vi "[BLE Test] ble_read_write_characteristics.vi"() -> ()   [LabVIEW 2015]
uses:
  Lib_Bled112 toolkit/type_def/connection_status_bundle.ctl
  Lib_Bled112 toolkit/type_def/address_type.ctl
  Lib_Bled112 toolkit/type_def/message_type.ctl
  Lib_Bled112 toolkit/type_def/message_class.ctl
  Lib_Bled112 toolkit/ble_functions/ble_write_by_handle_uint8array.vi
panel:
  out "Rx Packet Structure":T1={"Message Type (Response)"=128, "Payload length"=0, "Command Class (System)"=1, "Message ID"=0, "Connection handle"=0, "Attribute handle"=0, "Attribute type"=1, "Attribute value (data)"=[]} {"Attribute type" format="%02x" items=["read", "notify", "indicate", "read_by_type", "read_blob", "indicate_rsp_req"]; "Attribute value (data)" format="%02x"; "Attribute handle" format="%04x"; "Connection handle" format="%02x"; "Message ID" format="%02x"; "Message Type (Response)" format="%02x" items=["Command / Response"=0, "Event"=128]; "Command Class (System)" format="%02x" items=["System", "Persistent Store", "Attribute database", "Connection", "Attribute client", "Security Manager", "Generic Access Profile", "Hardware"]}
  out "Packet Detect":bool=TRUE
  out "Disconnected":bool=TRUE
  out "Scan success?":bool
  out "BLED112 Dongle Info":string="Major: 1, Minor: 3, Patch: 2, Build: 122, LL ver: 3, Protocol ver: 1 and HW ver: 3  "
  out "그래프 타이머 값 1":u32=9582380
  out "CDC(PCAP02) Graph":waveform(sgl)[](graph)=[{"t0"=timestamp(3554331896.4574084 s since 1904-01-01), "dt"=0.03, "Y"=[1.0007696]}, {"t0"=timestamp(3554331896.4574084 s since 1904-01-01), "dt"=0.03, "Y"=[1.0004687]}]
  out "Working Time(H:M:S)":string="00:01:58"
  out "ms 타이머 값 2":u32=9464045
  in  "Device List":i32(listbox)=2
  out "Rx packet Interval graph":u32(graph)=30
  in  "Program Exit":bool=TRUE
  out "부분배열 2":u8[](array[numeric])=[253, 79, 255, 49, 255, 79, 255, 60, 255, 209, 65, 123, 0, 0, 0, 0, 0, 0, 0, 0] format="%x"
  out "Data-IMU":dbl=-3.014375 format="%.10f"
  out "Hex-IMU":i16=-689 format="%x"
  out "웨이브폼 차트-IMU":dbl(graph)=-3.014375
  in  "Index-IMU ch.":u8(slide)=1 min=1 max=6 step=1 scale=1.0..6.0
  out "Rx OK":bool=TRUE
  out "ms 타이머 값":u32=9582439
  out "Entire-Rx time(ms)":i32=30
  in  "Index-CDC ch.":u8(slide)=1 min=1 max=6 step=1 scale=1.0..6.0
  out "웨이브폼 차트 - CDC":sgl(graph)=1.0007696
  out "Hex-CDC":u32=2098766 format="%x"
  out "Data-CDC":dbl=1.0007696151733398 format="%.10f"
  out "부분배열":u8[](array[numeric])=[32, 6, 78, 32, 3, 215, 32, 6, 110, 32, 71, 249, 32, 115, 92, 32, 30, 38, 1, 0] format="%x"
  in  "Tx 문자열":string="\nBLED112 Test\n"
  in  "Tx Send":bool
  out "Rx Cnt":i32=3775
  in  "Rx Stop":bool=TRUE
  out "Rx 문자열 1":string
  out "Connected":bool
  out "Device Name":string
  out "Address Type":enum16{"Public", "Random"}(ring)=enum."Random"
  out "Handle table":string[][](array[string])
  out "Connection Status":T4 {"Address Type" items=["Public", "Random"]}
  out "Scanning":bool
  in  "Device Connect":bool=TRUE
  out "MAC Address":string="D9:2F:10:92:34:F2"
  in  "COM Bluegiga in":refnum<visa-resource-name>="COM8"
  # "GEN4 1st PP - BLE(Bluetooth Low Energy) Test"
  # "CDC Data"
  # "SCAN"
  # "DEVICES FOUND"
  # "CONNECT"
  # "Introduce the MAC Address and Address Type of the device you want to connect and click in the CONTINUE button"
  # "IMU Data"
  # "Service 0x1800\nCharacteristic 0x2A00\nDevice Name"
  # "READING DEVICE NAME"
  # "Read"
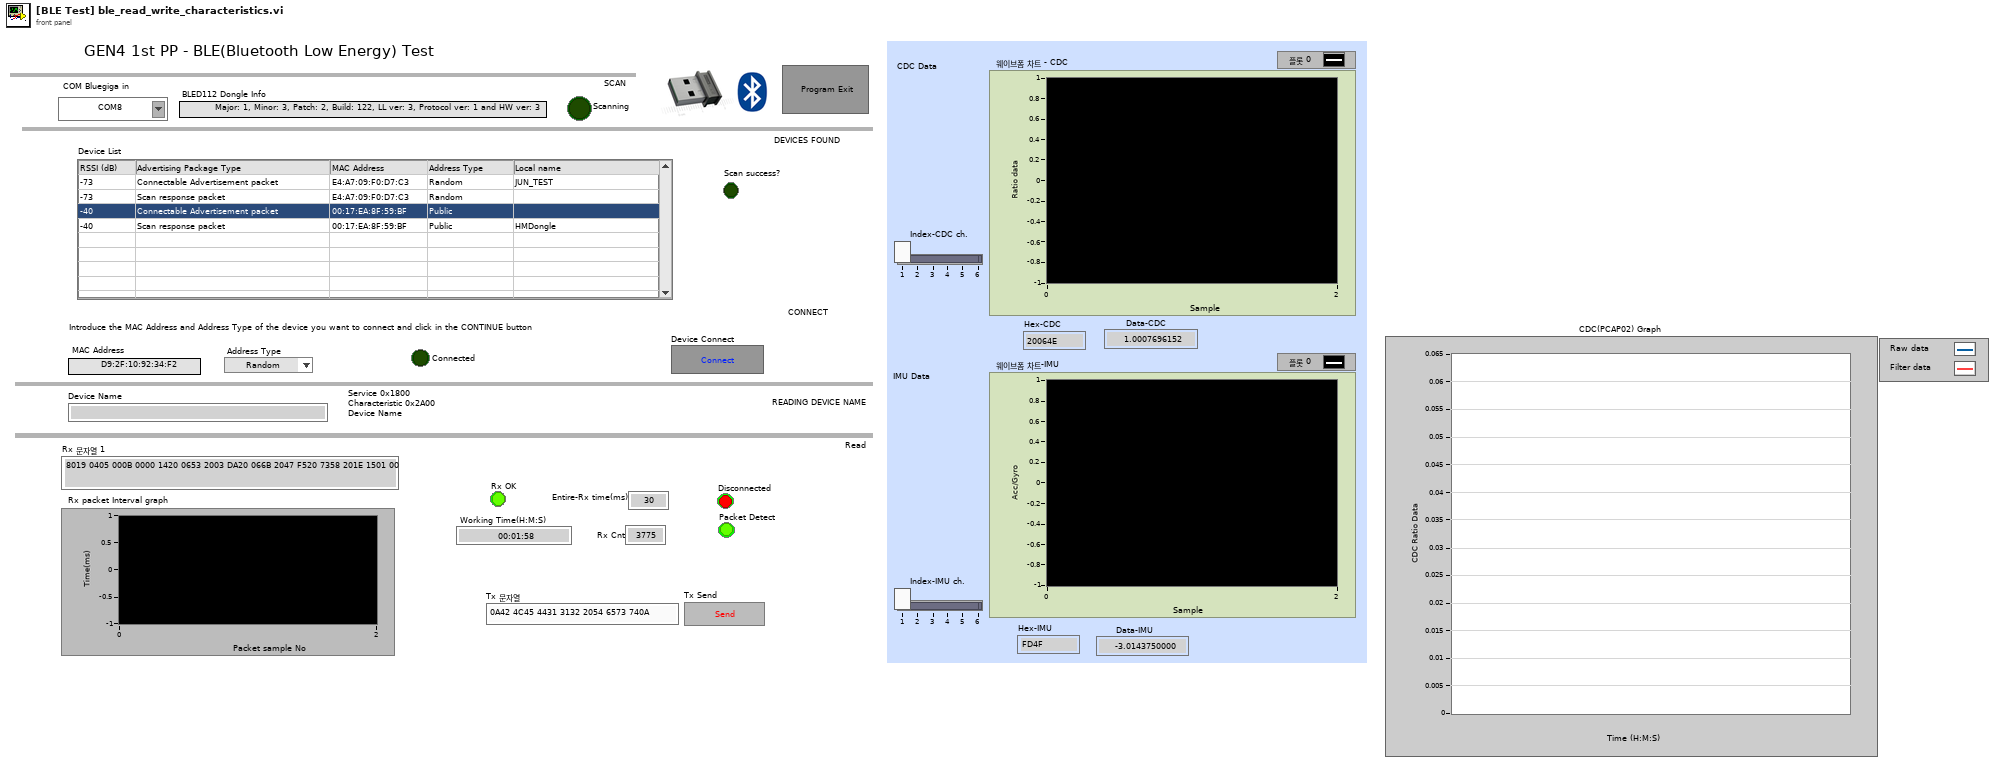
[diagram p1: front panel]
types:
  T1 = typedef "컨트롤-BLED Rx (EVENT-Attribute Client).ctl" = cluster{"Message Type (Response)":T2, "Payload length":u8, "Command Class (System)":T3, "Message ID":u8, "Connection handle":u8, "Attribute handle":u16, "Attribute type":T3, "Attribute value (data)":u8[]}
  T2 = typedef "message_type.ctl" = u8
  T3 = typedef "message_class.ctl" = u8
  T4 = typedef "connection_status_bundle.ctl" = cluster{"MAC Address":string, "cnx handle":u8, "cnx flags":u8, "Address Type":T5, "Connection Interval (ms)":u16, "Timeout(ms)":u16, "Latency":u16, "bonding handle":u8}
  T5 = typedef "address_type.ctl" = u8
  T6 = typedef "컨트롤-BLED Rx (EVENT-Connection status).ctl" = cluster{"Message Type (Response)":T2, "Payload length":u8, "Command Class (System)":T3, "Message ID":u8, "Connection handle":u8, "flags":u8, "Bluetooth address":u8[], "address type":T3, "conn_interval(ms)":dbl, "timeout(ms)":dbl, "latency":u16, "bonding(0xFF)":u8}
  T7 = typedef "컨트롤-BLED Rx (EVENT-Disconnected).ctl" = cluster{"Message Type (Response)":T2, "Payload length":u8, "Command Class (Connection)":T3, "Message ID":u8, "connection":u8, "reason":u16}
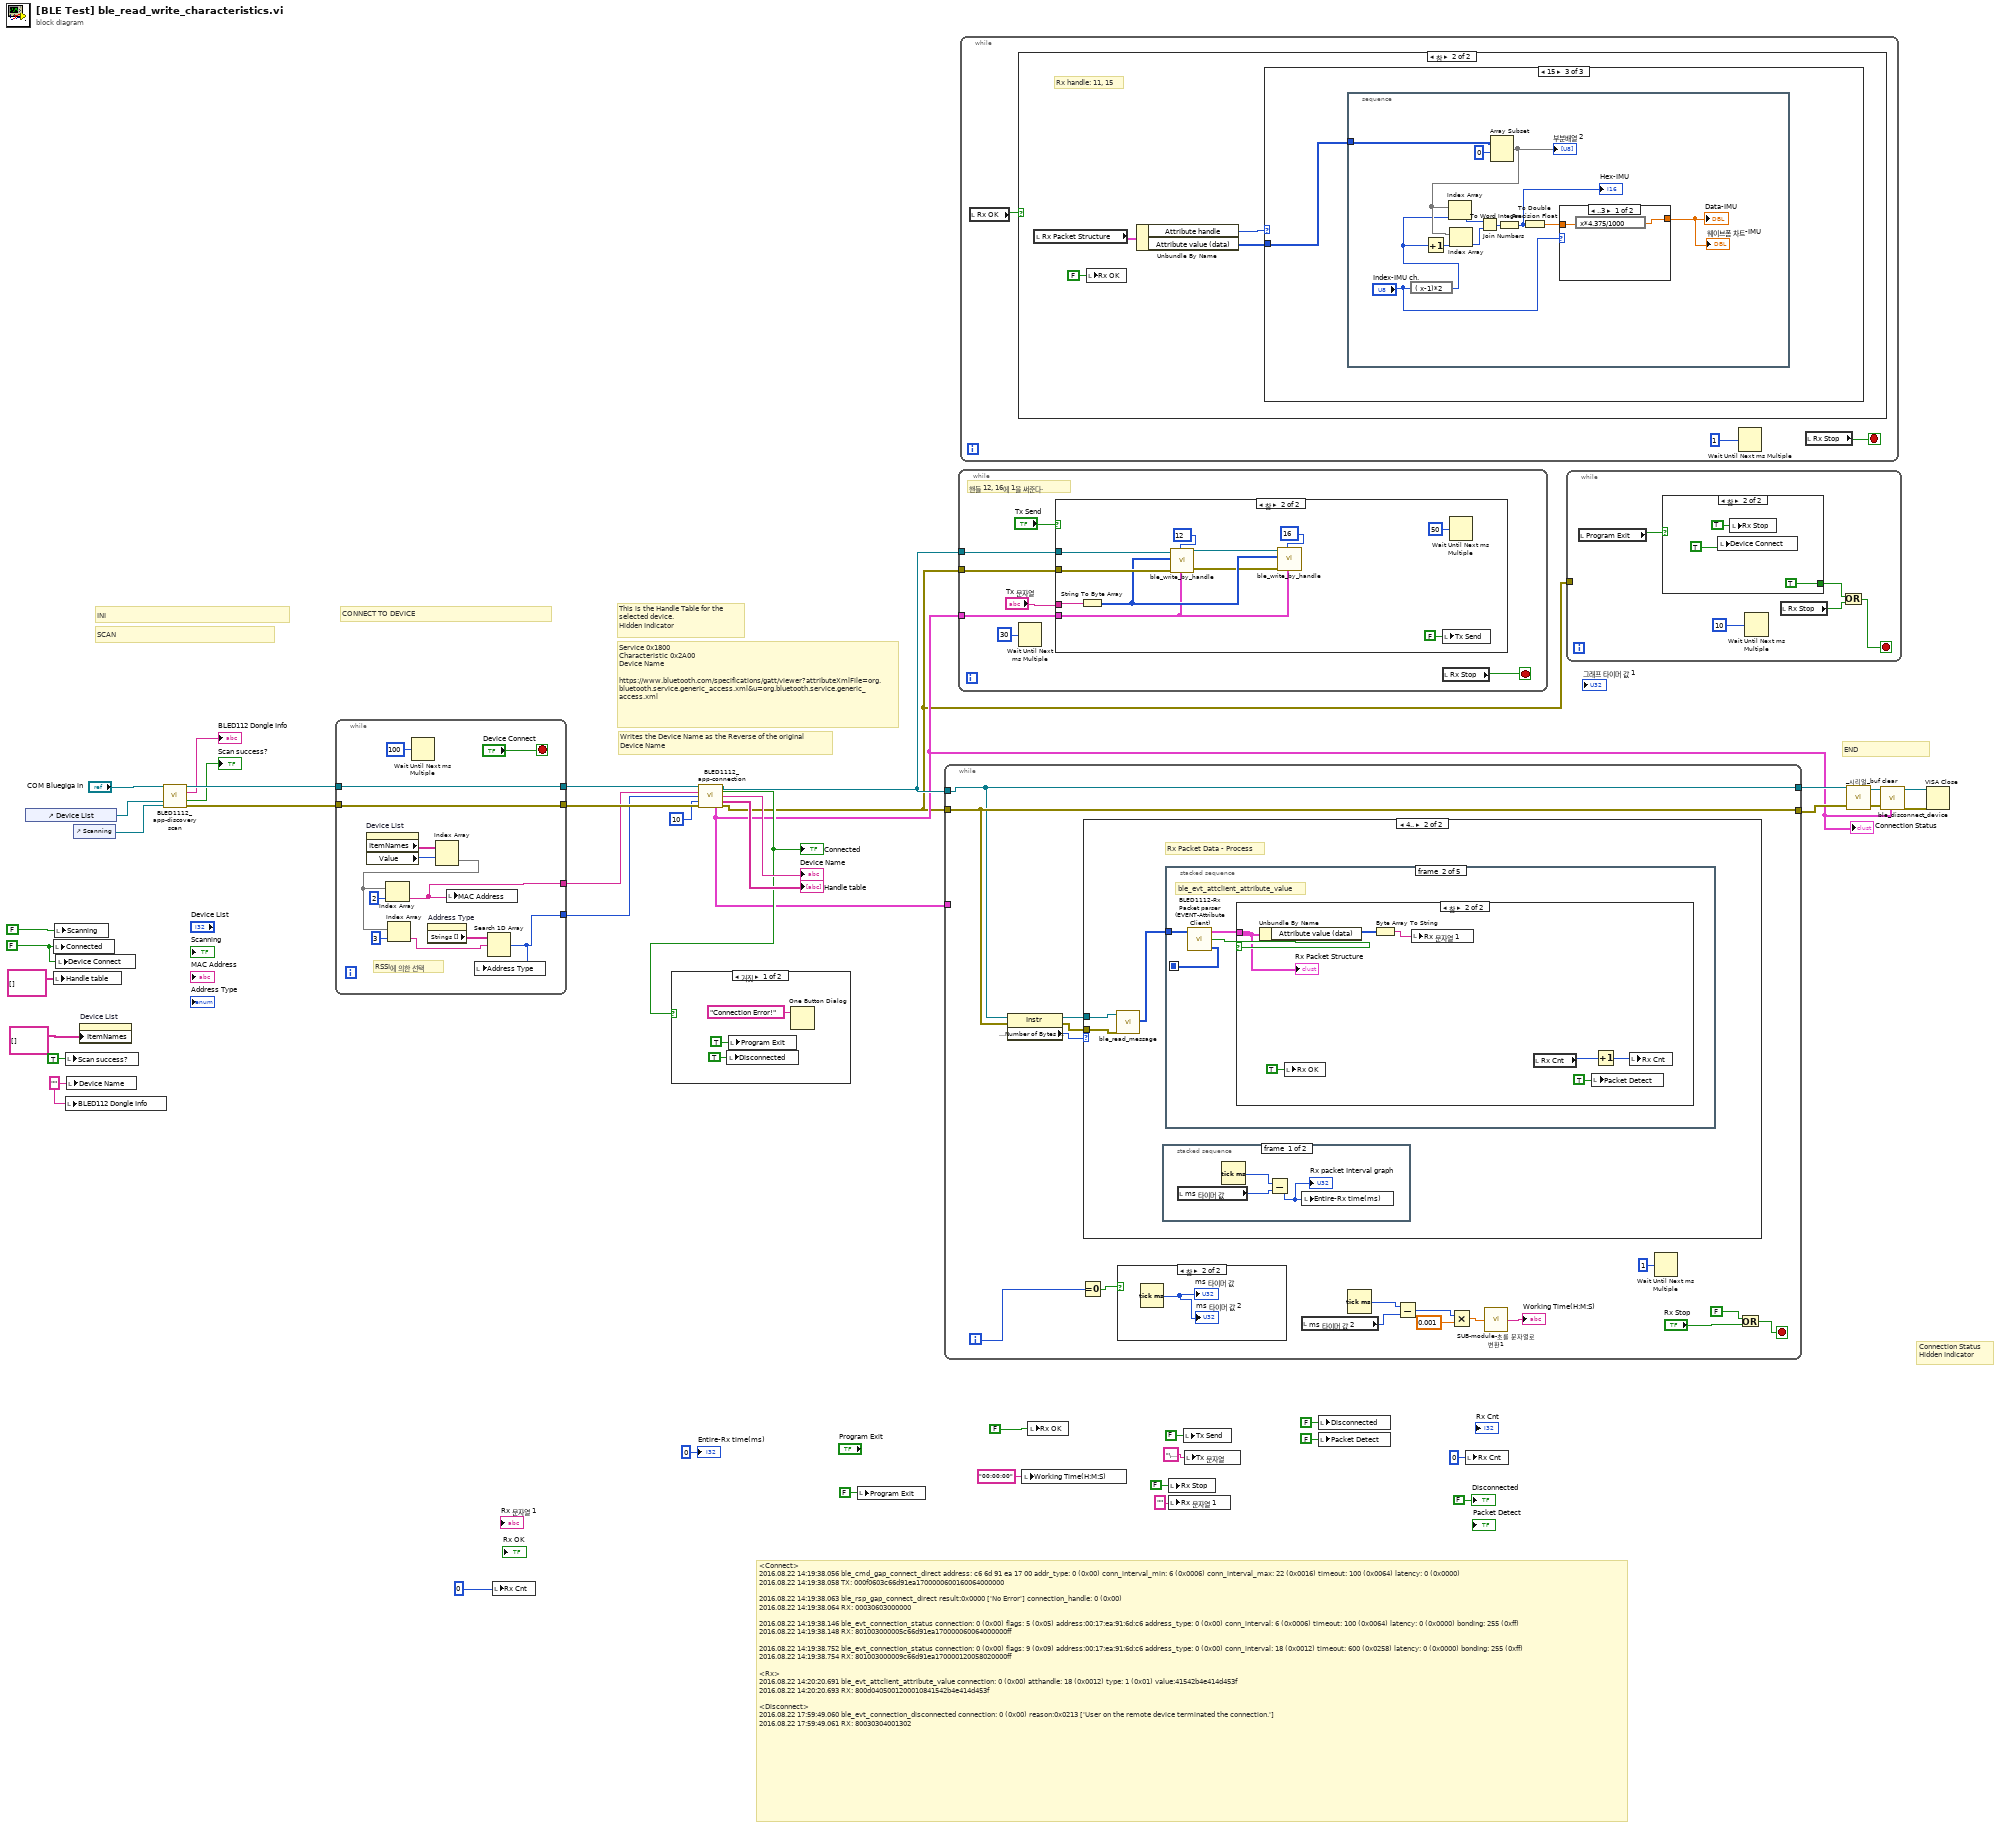
[diagram p0: block diagram]
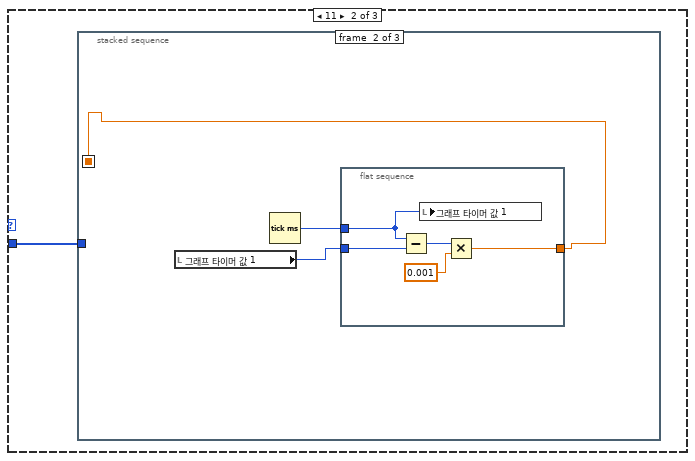
[diagram p7: hidden frame]
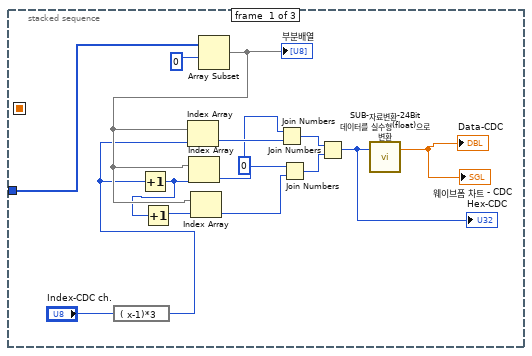
[diagram p8: hidden frame]
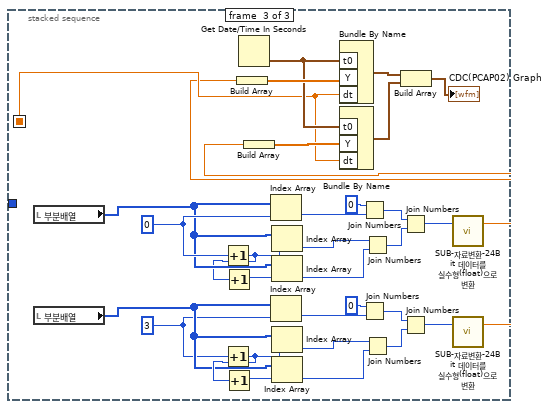
[diagram p9: hidden frame]
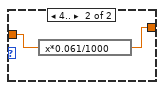
[diagram p10: hidden frame]
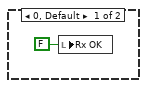
[diagram p11: hidden frame]
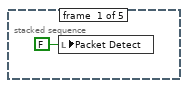
[diagram p12: hidden frame]
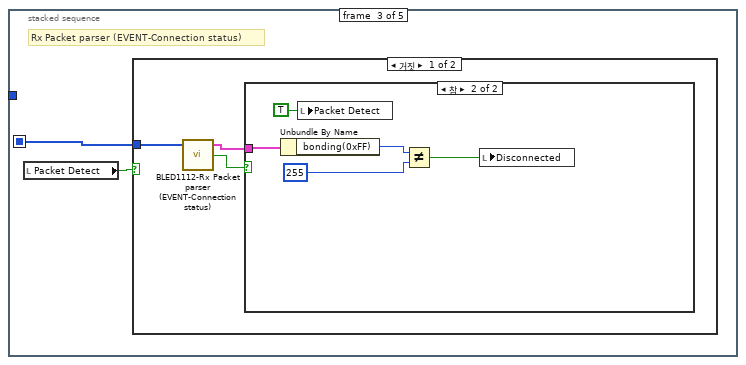
[diagram p14: hidden frame]
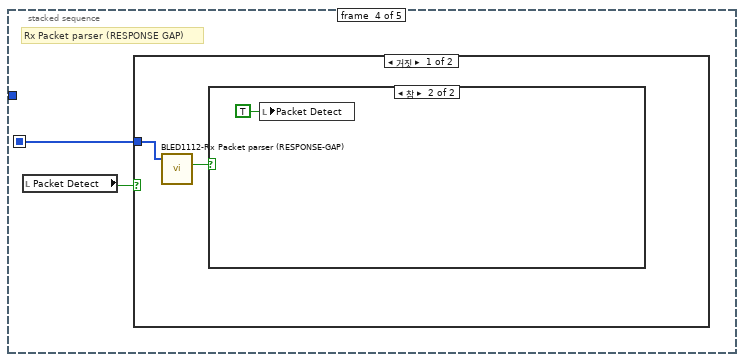
[diagram p17: hidden frame]
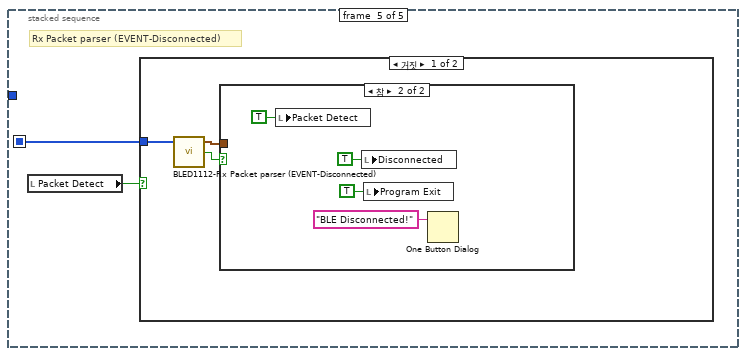
[diagram p20: hidden frame]
diagram:
  w19 = "" ("Device Name")
  w40 = FALSE ("Connected")
  # "<Connect>\n2016.08.22 14:19:38.056 ble_cmd_gap_connect_direct address: c6 6d 91 ea 17 00 addr_type: 0 (0x00) conn_interval_min: 6 (0x0006) conn_interval_max: 22 (0x0016) timeout: 100 (0x0064) latency: 0 (0x0000)\n2016.08.22 14:19:38.058 TX: 000f0603c66d91ea1700000600160064000000\n\n2016.08.22 14:19:38.063 ble_rsp_gap_connect_direct result:0x0000 ['No Error'] connection_handle: 0 (0x00)\n2016.08.22 14:19:38.064 RX: 00030603000000\n\n2016.08.22 14:19:38.146 ble_evt_connection_status connection: 0 (0x00) flags: 5 (0x05) address:00:17:ea:91:6d:c6 address_type: 0 (0x00) conn_interval: 6 (0x0006) timeout: 100 (0x0064) latency: 0 (0x0000) bonding: 255 (0xff)\n2016.08.22 14:19:38.148 RX: 801003000005c66d91ea170000060064000000ff\n\n2016.08.22 14:19:38.752 ble_evt_connection_status connection: 0 (0x00) flags: 9 (0x09) address:00:17:ea:91:6d:c6 address_type: 0 (0x00) conn_interval: 18 (0x0012) timeout: 600 (0x0258) latency: 0 (0x0000) bonding: 255 (0xff)\n2016.08.22 14:19:38.754 RX: 801003000009c66d91ea170000120058020000ff\n\n<Rx>\n2016.08.22 14:20:20.691 ble_evt_attclient_attribute_value connection: 0 (0x00) atthandle: 18 (0x0012) type: 1 (0x01) value:41542b4e414d453f\n2016.08.22 14:20:20.693 RX: 800d0405001200010841542b4e414d453f\n\n<Disconnect>\n2016.08.22 17:59:49.060 ble_evt_connection_disconnected connection: 0 (0x00) reason:0x0213 ['User on the remote device terminated the connection.']\n2016.08.22 17:59:49.061 RX: 80030304001302"
  # "Writes the Device Name as the Reverse of the original\nDevice Name"
  # "Service 0x1800\nCharacteristic 0x2A00\nDevice Name\n\nhttps://www.bluetooth.com/specifications/gatt/viewer?attributeXmlFile=org.bluetooth.service.generic_access.xml&u=org.bluetooth.service.generic_access.xml"
  # "This is the Handle Table for the\nselected device. \nHidden Indicator"
  # "Connection Status\nHidden Indicator"
  # "CONNECT TO DEVICE"
  # "SCAN"
  # "END"
  # "INI"
  n1 = control-ref of="Device List"() -> (w23:refnum<vi>)
  n2 = local write "Connected"(w40) -> ()
  n3 = local write "Handle table"(string[][] [] ("Handle table")) -> ()
  n4 = local write "Scanning"(FALSE ("Scanning")) -> ()
  n5 = local write "Device Connect"(w40) -> ()
  n6 = local write "Scan success?"(TRUE ("Scan success?")) -> ()
  n7 = local write "BLED112 Dongle Info"(w19) -> ()
  n8 = local write "Device Name"(w19) -> ()
  n9 = control-ref of="Scanning"() -> (w22:refnum<vi>)
  n10 = property on="Device List" class="MCListbox (엄격한)"("ItemNames"=string[][] [] ("Devices")) -> ()  [unwired: 2 in, 2 out]
  n11 = call "BLED1112_app-discovery scan.vi"("COM in"="COM Bluegiga in", "Device List"=w23, "LED ref"=w22) -> ("COM out"=w21:refnum<visa-resource-name>, "BLED112 Dongle Info"=→"BLED112 Dongle Info":string, "Scan success?"=→"Scan success?":bool, "error out"=w18:errorcluster)  [unwired: 8 in, 1 out]
  n12 = while {
    tunnel: w18 -> [w45]
    tunnel: [w55] -> w11
    tunnel: w21 -> [w55]
    tunnel: [w45] -> w10
    tunnel: [w51] -> w9
    tunnel: [w46] -> w8
    stop <- "Device Connect" stop-if-true
    # "RSSI에 의한 선택"
    n13 = property on="Device List" class="MCListbox (엄격한)"() -> ("ItemNames"=w54:string[][], "Value"=w53:i32)  [unwired: 2 in, 2 out]
    n14 = Wait Until Next ms Multiple(millisecond multiple=u32 100 ("ms 배수")) -> ()  [unwired: 1 out]
    n15 = property on="Address Type" class="Enum (엄격한)"() -> ("Strings []"=w48:string[])  [unwired: 2 in, 2 out]
    n16 = Index Array(array=w54, index (row)=w53) -> (element=w49:string[])  [unwired: 1 in]
    n17 = Index Array(array=w49, index=2 ("인덱스")) -> (element=w51:string)
    n18 = Index Array(array=w49, index=3 ("인덱스")) -> (element=w47:string)
    n19 = local write "MAC Address"(w51) -> ()
    n20 = Search 1D Array(1D array=w48, element=w47) -> (index of element=w46:i32)  [unwired: 1 in]
    n21 = local write "Address Type"(w46) -> ()
  }
  n22 = local write "Rx Cnt"(u32 0 ("CDC-Rx time(ms)")) -> ()
  n23 = call "BLED1112_app-connection.vi"("COM Bluegiga in"=w11, "MAC Address"=w9, "Address Type"=w8, "Conn Try no"=10, "error in"=w10) -> ("COM out"=w7:refnum<visa-resource-name>, "Connection Ok"=w3:bool, "Device Name"=→"Device Name":string, "Handle table"=→"Handle table":string[][], "Connection Status"=w2:T4, "에러 출력"=w1:errorcluster)  [unwired: 5 in]
  "Connection Status" <- w2
  "Connected" <- w3
  n24 = case shown="거짓" w3 {
    frame False {
      n25 = local write "Disconnected"(TRUE ("Disconnected")) -> ()
      n26 = local write "Program Exit"(TRUE ("정지")) -> ()
      n27 = One Button Dialog(message="Connection Error!" ("메시지")) -> ()  [unwired: 1 in, 1 out]
    }
    frame True {
    }
  }
  n28 = local write "Program Exit"(FALSE ("정지")) -> ()
  n29 = while {
    tunnel: w7 -> [w63]
    tunnel: w1 -> [w64]
    tunnel: w2 -> [_]
    tunnel: [w63] -> w38
    tunnel: [w64] -> w37
    i -> [w74]
    stop <- w75 stop-if-true
    n30 = property class="Instr"(reference=w63, error in=w64) -> (reference out=w61:refnum<visa-resource-name>, error out=w60:errorcluster, "Serial Settings:Number of Bytes at Serial Port"=w62:u32)
    n31 = Equal To 0?(x=w74) -> (x = 0?=w73:bool)
    n32 = case shown="4.." w62 {
      tunnel: w61 -> [_ w80]
      tunnel: w60 -> [_ w79]
      frame 0, Default {
        n33 = local write "Rx OK"(FALSE ("Rx OK")) -> ()
      }
      frame 4.. {
        # "Rx Packet Data - Process"
        n34 = call "ble_read_message.vi"("error in (no error)"=w79, "COM Bluegiga in"=w80) -> ("message package"=w78:u8[])  [unwired: 7 in, 2 out]
        n35 = stacked-sequence {
          frame #0 {
            n36 = local read "ms 타이머 값"() -> (w119:u32)
            n37 = Tick Count (ms)() -> (millisecond timer value=w118:u32)
            n38 = Subtract(x=w118, y=w119) -> (x-y=w117:u32)
            "Rx packet Interval graph" <- w117
            n39 = local write "Entire-Rx time(ms)"(w117) -> ()
          }
          frame #1 {
            n40 = Tick Count (ms)() -> (millisecond timer value=w120:u32)
            n41 = local write "ms 타이머 값"(w120) -> ()
          }
        }
        n42 = stacked-sequence {
          seq-local: [_ w84 _ _ _] -> [_ _ w94 w104 w109]
          tunnel: w78 -> [_ w85 _ _ _]
          frame #0 {
            n43 = local write "Packet Detect"(FALSE ("Packet Detect")) -> ()
          }
          frame #1 {
            # "ble_evt_attclient_attribute_value"
            n44 = call "BLED1112-Rx Packet parser (EVENT-Attribute Client).vi"("message package"=w85) -> ("message out"=w84:u8[], "Packet OK"=w83:bool, "Data Structure"=w82:T1)  [unwired: 2 in]
            n45 = case shown="참" w83 {
              tunnel: w82 -> [_ w90]
              frame False {
              }
              frame True {
                n46 = Unbundle By Name(w90) -> ("Attribute value (data)"=w88:u8[])
                n47 = local write "Rx OK"(TRUE ("Rx OK")) -> ()
                n48 = Byte Array To String(unsigned byte array=w88) -> (string=w89:string)
                n49 = local write "Rx 문자열 1"(w89) -> ()
                n50 = local read "Rx Cnt"() -> (w91:i32)
                n51 = local write "Packet Detect"(TRUE ("Packet Detect")) -> ()
                n52 = Increment(x=w91) -> (x+1=w92:i32)
                n53 = local write "Rx Cnt"(w92) -> ()
                "Rx Packet Structure" <- w90
              }
            }
          }
          frame #2 {
            # "Rx Packet parser (EVENT-Connection status)"
            n54 = local read "Packet Detect"() -> (w93:bool)
            n55 = case shown="거짓" w93 {
              tunnel: w94 -> [w97 _]
              frame False {
                n56 = call "BLED1112-Rx Packet parser (EVENT-Connection status).vi"("message package"=w97) -> ("Packet OK"=w96:bool, "Data Structure"=w95:T6)  [unwired: 2 in, 1 out]
                n57 = case shown="참" w96 {
                  tunnel: w95 -> [_ w102]
                  frame False {
                  }
                  frame True {
                    n58 = Unbundle By Name(w102) -> ("bonding(0xFF)"=w101:u8)
                    n59 = local write "Packet Detect"(TRUE ("Packet Detect")) -> ()
                    n60 = Not Equal?(x=w101, y=255 ("Rx Cnt")) -> (x != y?=w99:bool)
                    n61 = local write "Disconnected"(w99) -> ()
                  }
                }
              }
              frame True {
              }
            }
          }
          frame #3 {
            # "Rx Packet parser (RESPONSE GAP)"
            n62 = local read "Packet Detect"() -> (w103:bool)
            n63 = case shown="거짓" w103 {
              tunnel: w104 -> [w106 _]
              frame False {
                n64 = call "BLED1112-Rx Packet parser (RESPONSE-GAP).vi"("message package"=w106) -> ("Packet OK"=w105:bool)  [unwired: 2 in, 2 out]
                n65 = case shown="참" w105 {
                  frame False {
                  }
                  frame True {
                    n66 = local write "Packet Detect"(TRUE ("Packet Detect")) -> ()
                  }
                }
              }
              frame True {
              }
            }
          }
          frame #4 {
            # "Rx Packet parser (EVENT-Disconnected)"
            n67 = local read "Packet Detect"() -> (w108:bool)
            n68 = case shown="거짓" w108 {
              tunnel: w109 -> [w111 _]
              frame False {
                n69 = call "BLED1112-Rx Packet parser (EVENT-Disconnected).vi"("message package"=w111) -> ("Packet OK"=w112:bool, "Data Structure"=w110:T7)  [unwired: 2 in, 1 out]
                n70 = case shown="참" w112 {
                  tunnel: w110 -> [_ _]
                  frame False {
                  }
                  frame True {
                    n71 = local write "Packet Detect"(TRUE ("Packet Detect")) -> ()
                    n72 = local write "Disconnected"(TRUE ("Disconnected")) -> ()
                    n73 = local write "Program Exit"(TRUE ("정지")) -> ()
                    n74 = One Button Dialog(message="BLE Disconnected!" ("메시지")) -> ()  [unwired: 1 in, 1 out]
                  }
                }
              }
              frame True {
              }
            }
          }
        }
      }
    }
    n75 = case shown="참" w73 {
      frame False {
      }
      frame True {
        n76 = Tick Count (ms)() -> (millisecond timer value=→"ms 타이머 값" →"ms 타이머 값 2":u32)
      }
    }
    n77 = local read "ms 타이머 값 2"() -> (w71:u32)
    n78 = Tick Count (ms)() -> (millisecond timer value=w72:u32)
    n79 = Subtract(x=w72, y=w71) -> (x-y=w68:u32)
    n80 = Multiply(x=w68, y=0.001) -> (x*y=w70:dbl)
    n81 = call "SUB-module-초를 문자열로 변환1.vi"("입력-초단위"=w70) -> ("시:분:초"=→"Working Time(H:M:S)":string)
    n82 = Wait Until Next ms Multiple(millisecond multiple=u32 1 ("ms 배수")) -> ()  [unwired: 1 out]
    n83 = Or(x=FALSE, y="Rx Stop") -> (x .or. y?=w75:bool)
  }
  n84 = while {
    tunnel: w7 -> [w125]
    tunnel: w1 -> [w124]
    tunnel: w2 -> [w122]
    stop <- w126 stop-if-true
    # "핸들 12, 16에 1을 써준다."
    n85 = Wait Until Next ms Multiple(millisecond multiple=u32 30 ("ms 배수")) -> ()  [unwired: 1 out]
    n86 = case shown="참" "Tx Send" {
      tunnel: w125 -> [_ w139]
      tunnel: w124 -> [_ w138]
      tunnel: "Tx 문자열" -> [_ w133]
      tunnel: w122 -> [_ w129]
      frame False {
      }
      frame True {
        n87 = String To Byte Array(string=w133) -> (unsigned byte array=w132:u8[])
        n88 = call-poly "ble_write_by_handle.vi"("Connection Status"=w129, "Handle"=u16 12, "error in (no error)"=w138, "data (uint8array)"=w132, "COM Bluegiga in"=w139) -> ("error out"=w130:errorcluster, "COM Bluegiga out"=w131:refnum<visa-resource-name>)  [unwired: 5 in]
        n89 = call-poly "ble_write_by_handle.vi"("Connection Status"=w129, "Handle"=u16 16, "error in (no error)"=w130, "data (uint8array)"=w132, "COM Bluegiga in"=w131) -> ()  [unwired: 5 in, 2 out]
        n90 = local write "Tx Send"(FALSE ("Tx Send")) -> ()
        n91 = Wait Until Next ms Multiple(millisecond multiple=u32 50 ("ms 배수")) -> ()  [unwired: 1 out]
      }
    }
    n92 = local read "Rx Stop"() -> (w126:bool)
  }
  n93 = while {
    stop <- w142 stop-if-true
    n94 = local read "Rx OK"() -> (w140:bool)
    n95 = case shown="참" w140 {
      frame False {
      }
      frame True {
        # "Rx handle: 11, 15"
        n96 = local read "Rx Packet Structure"() -> (w146:T1)
        n97 = local write "Rx OK"(FALSE ("Rx OK")) -> ()
        n98 = Unbundle By Name(w146) -> ("Attribute handle"=w145:u16, "Attribute value (data)"=w143:u8[])
        n99 = case shown="15" w145 {
          tunnel: w143 -> [_ w147 w202]
          frame 0, Default {
          }
          frame 11 {
            n100 = stacked-sequence {
              seq-local: [_ w163 _] -> [_ _ w195]
              tunnel: w147 -> [w148 _ _]
              frame #0 {
                n101 = expression code="( x-1)*3"("Index-CDC ch.") -> (w151:u8)
                n102 = Increment(x=w151) -> (x+1=w150:u8)
                n103 = Increment(x=w150) -> (x+1=w149:u8)
                n104 = Array Subset(array=w148, index=0 ("인덱스")) -> (w161:u8[])  [unwired: 1 in]
                "부분배열" <- w161
                n105 = Index Array(array=w161, index=w151) -> (element=w158:u8)
                n106 = Index Array(array=w161, index=w150) -> (element=w159:u8)
                n107 = Index Array(array=w161, index=w149) -> (element=w160:u8)
                n108 = Join Numbers(hi=u8 0 ("인덱스"), lo=w158) -> ((hi.lo)=w155:u16)
                n109 = Join Numbers(hi=w159, lo=w160) -> ((hi.lo)=w156:u16)
                n110 = Join Numbers(hi=w155, lo=w156) -> ((hi.lo)=w154:u32)
                "Hex-CDC" <- w154
                n111 = call "SUB-자료변환-24Bit 데이터를 실수형(float)으로 변환.vi"("U32"=w154) -> ("FP32"=→"Data-CDC" →"웨이브폼 차트 - CDC":sgl)  [unwired: 2 in]
              }
              frame #1 {
                n112 = local read "그래프 타이머 값 1"() -> (w165:u32)
                n113 = Tick Count (ms)() -> (millisecond timer value=w164:u32)
                n114 = flat-sequence {
                  tunnel: w164 -> [w170]
                  tunnel: w165 -> [w167]
                  tunnel: [w166] -> w163
                  frame #0 {
                    n115 = Subtract(x=w170, y=w167) -> (x-y=w168:u32)
                    n116 = local write "그래프 타이머 값 1"(w170) -> ()
                    n117 = Multiply(x=w168, y=0.001 ("dt")) -> (x*y=w166:dbl)
                  }
                }
              }
              frame #2 {
                w173 = u8 3 ("인덱스")
                w194 = u8 0 ("인덱스")
                n118 = local read "부분배열"() -> (w193:u8[])
                n119 = local read "부분배열"() -> (w174:u8[])
                n120 = Increment(x=w194) -> (x+1=w185:u8)
                n121 = Increment(x=w173) -> (x+1=w182:u8)
                n122 = Increment(x=w185) -> (x+1=w184:u8)
                n123 = Increment(x=w182) -> (x+1=w183:u8)
                n124 = Get Date/Time In Seconds() -> (seconds since 1Jan1904=w199:timestamp)
                n125 = Index Array(array=w193, index=w194) -> (element=w190:u8)
                n126 = Index Array(array=w174, index=w173) -> (element=w177:u8)
                n127 = Index Array(array=w193, index=w185) -> (element=w191:u8)
                n128 = Index Array(array=w193, index=w184) -> (element=w192:u8)
                n129 = Index Array(array=w174, index=w182) -> (element=w176:u8)
                n130 = Index Array(array=w174, index=w183) -> (element=w175:u8)
                n131 = Join Numbers(hi=u8 0 ("인덱스"), lo=w190) -> ((hi.lo)=w187:u16)
                n132 = Join Numbers(hi=u8 0 ("인덱스"), lo=w177) -> ((hi.lo)=w180:u16)
                n133 = Join Numbers(hi=w191, lo=w192) -> ((hi.lo)=w188:u16)
                n134 = Join Numbers(hi=w176, lo=w175) -> ((hi.lo)=w179:u16)
                n135 = Join Numbers(hi=w187, lo=w188) -> ((hi.lo)=w186:u32)
                n136 = Join Numbers(hi=w180, lo=w179) -> ((hi.lo)=w181:u32)
                n137 = call "SUB-자료변환-24Bit 데이터를 실수형(float)으로 변환.vi"("U32"=w186) -> ("FP32"=w172:sgl)  [unwired: 2 in]
                n138 = Build Array(w172) -> (w200:sgl[])
                n139 = Bundle By Name("t0"=w199, "Y"=w200, "dt"=w195) -> (w196:waveform(sgl))  [unwired: 1 in]
                n140 = call "SUB-자료변환-24Bit 데이터를 실수형(float)으로 변환.vi"("U32"=w181) -> ("FP32"=w171:sgl)  [unwired: 2 in]
                n141 = Build Array(w171) -> (w201:sgl[])
                n142 = Bundle By Name("t0"=w199, "Y"=w201, "dt"=w195) -> (w197:waveform(sgl))  [unwired: 1 in]
                n143 = Build Array(w196, w197) -> (→"CDC(PCAP02) Graph":waveform(sgl)[])
              }
            }
          }
          frame 15 {
            n144 = stacked-sequence {
              tunnel: w202 -> [w203]
              frame #0 {
                n145 = expression code="( x-1)*2"("Index-IMU ch.") -> (w207:u8)
                n146 = Increment(x=w207) -> (x+1=w206:u8)
                n147 = Array Subset(array=w203, index=0 ("인덱스")) -> (w213:u8[])  [unwired: 1 in]
                "부분배열 2" <- w213
                n148 = Index Array(array=w213, index=w207) -> (element=w212:u8)
                n149 = Index Array(array=w213, index=w206) -> (element=w211:u8)
                n150 = Join Numbers(hi=w212, lo=w211) -> ((hi.lo)=w209:u16)
                n151 = To Word Integer(number=w209) -> (16bit integer=w205:i16)
                "Hex-IMU" <- w205
                n152 = To Double Precision Float(number=w205) -> (double precision float=w208:dbl)
                n153 = case shown="..3" "Index-IMU ch." {
                  tunnel: [w216 w217] -> w210
                  tunnel: w208 -> [w215 w218]
                  frame ..3 {
                    n154 = expression code="x*4.375/1000"(w215) -> (w216:dbl)
                  }
                  frame 4.. {
                    n155 = expression code="x*0.061/1000"(w218) -> (w217:dbl)
                  }
                }
                "Data-IMU" <- w210
                "웨이브폼 차트-IMU" <- w210
              }
            }
          }
        }
      }
    }
    n156 = Wait Until Next ms Multiple(millisecond multiple=u32 1 ("ms 배수")) -> ()  [unwired: 1 out]
    n157 = local read "Rx Stop"() -> (w142:bool)
  }
  n158 = local write "Working Time(H:M:S)"("00:00:00" ("Working Time(H:M:S)")) -> ()
  n159 = local write "Rx OK"(FALSE ("success?")) -> ()
  n160 = local write "Rx Stop"(FALSE ("Rx 정지")) -> ()
  n161 = local write "Rx 문자열 1"("" ("Rx 문자열")) -> ()
  n162 = local write "Tx Send"(FALSE ("Tx Send")) -> ()
  n163 = local write "Tx 문자열"("\u0001" ("Tx 문자열")) -> ()
  n164 = local write "Disconnected"(FALSE ("Disconnected")) -> ()
  n165 = local write "Packet Detect"(FALSE ("Packet Detect")) -> ()
  n166 = local write "Rx Cnt"(0 ("Rx Cnt")) -> ()
  n167 = while {
    tunnel: w1 -> [_]
    stop <- w219 stop-if-true
    n168 = local read "Program Exit"() -> (w223:bool)
    n169 = case shown="참" w223 {
      tunnel: [_ TRUE] -> w220
      frame False {
      }
      frame True {
        n170 = local write "Device Connect"(TRUE ("Continue")) -> ()
        n171 = local write "Rx Stop"(TRUE ("Rx 정지")) -> ()
      }
    }
    n172 = Wait Until Next ms Multiple(millisecond multiple=u32 10 ("ms 배수")) -> ()  [unwired: 1 out]
    n173 = local read "Rx Stop"() -> (w221:bool)
    n174 = Or(x=w220, y=w221) -> (x .or. y?=w219:bool)
  }
  n175 = call "_시리얼_buf clear.vi"("에러 출력 2"=w37, "시리얼 포트"=w38) -> ("에러 출력"=w26:errorcluster, "시리얼 포트 2"=w25:refnum<visa-resource-name>)  [unwired: 2 in]
  n176 = call "ble_disconnect_device.vi"("Connection Status"=w2, "error in (no error)"=w26, "COM Bluegiga in"=w25) -> ("error out"=w42:errorcluster, "COM Bluegiga out"=w43:refnum<visa-resource-name>)  [unwired: 7 in]
  n177 = VISA Close(VISA resource name=w43, error in (no error)=w42) -> ()  [unwired: 1 out]
  "Entire-Rx time(ms)" <- 0 ("수신 주기(ms)")
  "Disconnected" <- FALSE ("packer Parser")
